vi "Test Basic Read.vi"(8 "error in (no error)":errorcluster, 11 "Scalar Channels Testing in":refnum<class "Scalar Channels Testing.lvclass">) -> (0 "error out":errorcluster, 3 "Scalar Channels Testing out":refnum<class "Scalar Channels Testing.lvclass">)   [LabVIEW 2019, in "Scalar Channels Testing.lvclass"]
uses:
  Scalar Channels Testing.lvclass
  C:/Program Files (x86)/National Instruments/LabVIEW 2019/vi.lib/NI/NI VeriStand Development Tools/NI Veristand Test Utilities/VeriStandTestCase/VeriStandTestCase.lvclass
  <vilib>/NI VeriStand/Execution/Workspace/NI VeriStand - Get Single Channel Value.vi
  <vilib>/NI VeriStand/Execution/Workspace/NI_VS Workspace ExecutionAPI.lvlib
panel:
  out "Value":dbl
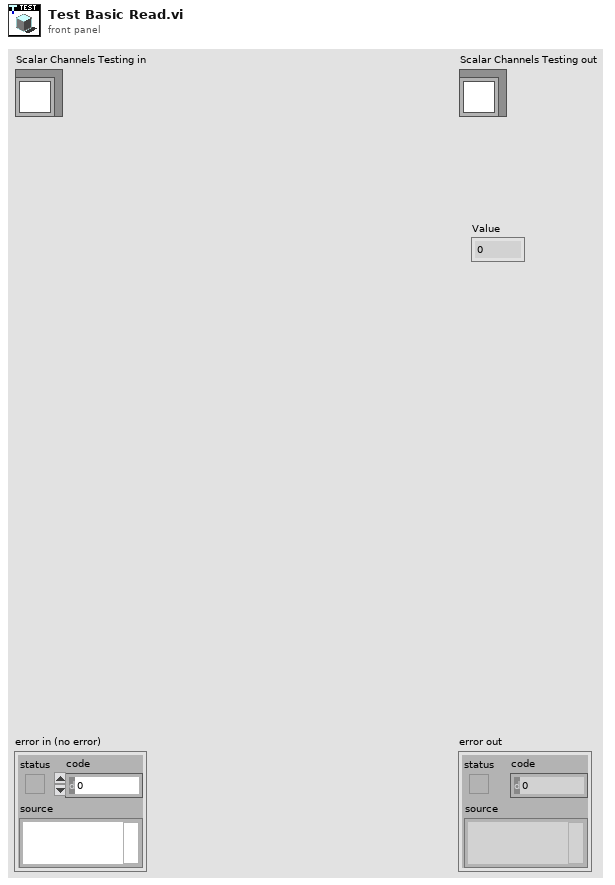
[diagram p1: front panel]
types:
  T1 = typedef "NI_VS Workspace ExecutionAPI.lvlib/WorkspaceAPI.ctl" = refnum<k24>
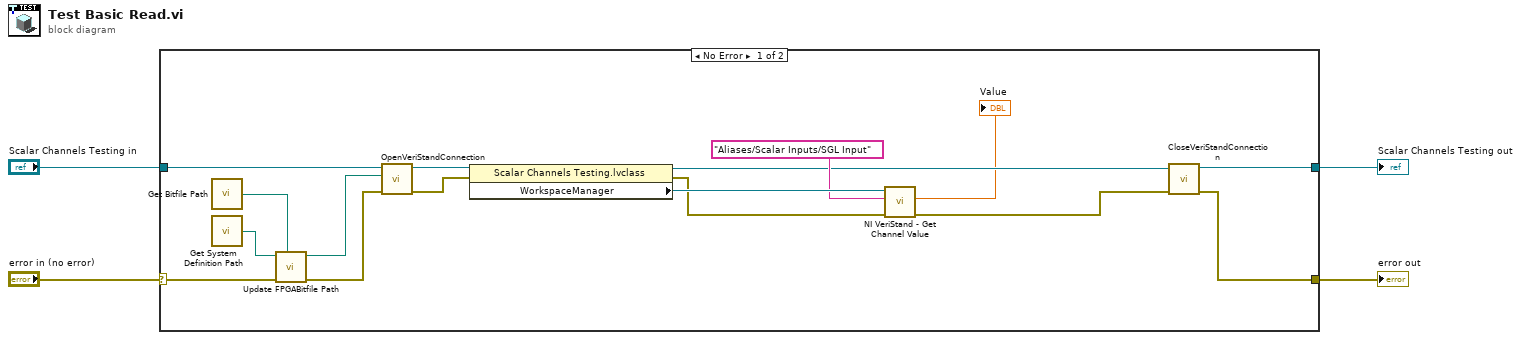
[diagram p0: block diagram]
diagram:
  n1 = case shown="No Error" "error in (no error)" {
    selector: "error in (no error)" -> [w7 w22]
    tunnel: [w18 w22] -> w3
    tunnel: [w19 w21] -> w1
    tunnel: "Scalar Channels Testing in" -> [w20 w21]
    frame No Error {
      n2 = call "Get Bitfile Path.vi"() -> ("Bitfile Path"=w9:path)
      n3 = call "Get System Definition Path.vi"() -> ("System Definition path"=w8:path)
      n4 = call "Update FPGABitfile Path.vi"("Bitfile Path"=w9, "error in (no error)"=w7, "System Definition path in"=w8) -> ("error out"=w6:errorcluster, "System Definition path out"=w5:path)  [unwired: 7 in]
      n5 = call-dynamic "OpenVeriStandConnection.vi"("error in (no error)"=w6, "System Definition File"=w5, "VeriStand Test Case in"=w20) -> ("error out"=w16:errorcluster, "VeriStand Test Case out"=w17:refnum<class "Scalar Channels Testing.lvclass">)  [unwired: 6 in, 1 out]
      n6 = property class="Scalar Channels Testing.lvclass"(reference=w17, error in=w16) -> (reference out=w13:refnum<class "Scalar Channels Testing.lvclass">, error out=w12:errorcluster, "WorkspaceManager"=w15:T1)
      n7 = call-poly <vilib>:"NI VeriStand - Get Channel Value.vi"("error in (no error)"=w12, "Channel"="Aliases/Scalar Inputs/SGL Input", "WorkspaceManager in"=w15) -> ("error out"=w11:errorcluster, "Value"=→"Value":dbl)  [unwired: 6 in, 1 out]
      n8 = call-dynamic "CloseVeriStandConnection.vi"("error in (no error)"=w11, "VeriStand Test Case in"=w13) -> ("error out"=w18:errorcluster, "VeriStand Test Case out"=w19:refnum<class "Scalar Channels Testing.lvclass">)  [unwired: 8 in]
    }
    frame Error {
    }
  }
  "error out" <- w3
  "Scalar Channels Testing out" <- w1
